vi "set Packet Timeout M Sec.vi"(10 "msec":dbl, 11 "port_num":i32) -> ()   [LabVIEW 2015, in "dxl_x86_c.lvlib"]
doc: "WINDECLSPEC void setPacketTimeoutMSec (int port_num, double msec);"
uses:
  dxl_x86_c.lvlib
  dxl_x86_c.dll
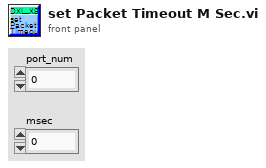
[diagram p1: front panel]
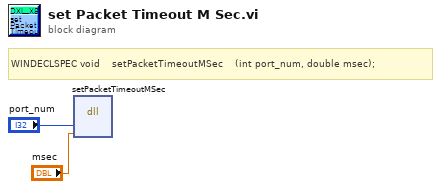
[diagram p0: block diagram]
diagram:
  # "WINDECLSPEC void    setPacketTimeoutMSec    (int port_num, double msec);"
  n1 = dll-call lib="C:/Users/Platform/Desktop/LabVIEW/dxl_x86_c.lvlib/dxl_x86_c.*" fn="setPacketTimeoutMSec"("port_num"="port_num", "msec"="msec") -> ()  [unwired: 6 in, 2 out]
